vi "Return Black Start Status.vi"(4 "Status":T1, 6 "error":string, 8 "error in (no error)":errorcluster, 10 "IED Name":string, 11 "SCADA in":refnum<class "SCADA.lvclass">) -> (0 "error out":errorcluster, 3 "SCADA out":refnum<class "SCADA.lvclass">)   [LabVIEW 2015, in "SCADA Core.lvlib" / "SCADA.lvclass"]
uses:
  SCADA.lvclass
  SCADA Abstract Messages/Black Start Status Msg/Black Start Status.ctl
  SCADA.lvclass/SCADA.ctl
  <vilib>/ActorFramework/Actor/Actor.lvclass/Actor.ctl
  Controls/Grid Mode.ctl
  <vilib>/ActorFramework/Actor/Actor.lvclass
  SCADA Abstract Messages/Black Start Status Msg/Black Start Status Msg.lvclass
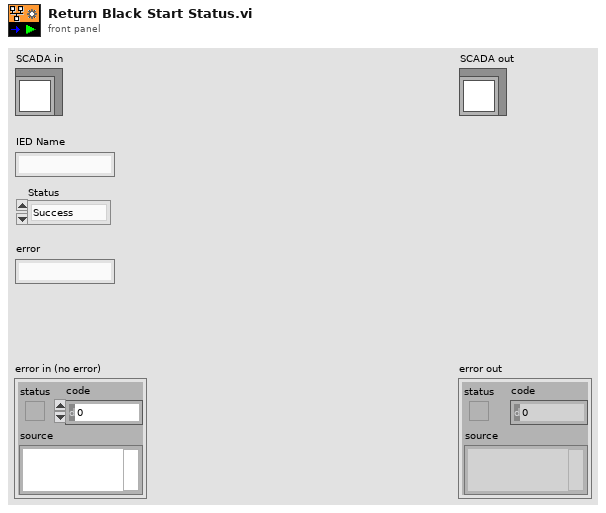
[diagram p1: front panel]
types:
  T1 = typedef "SCADA Core.lvlib/Black Start Status Msg.lvclass/Black Start Status.ctl" = enum16{"Success", "Failure"}
  T2 = typedef "SCADA Core.lvlib/SCADA.lvclass/Grid Mode.ctl" = enum16{"Off", "Grid Connected", "Islanded", "Synchronizing"}
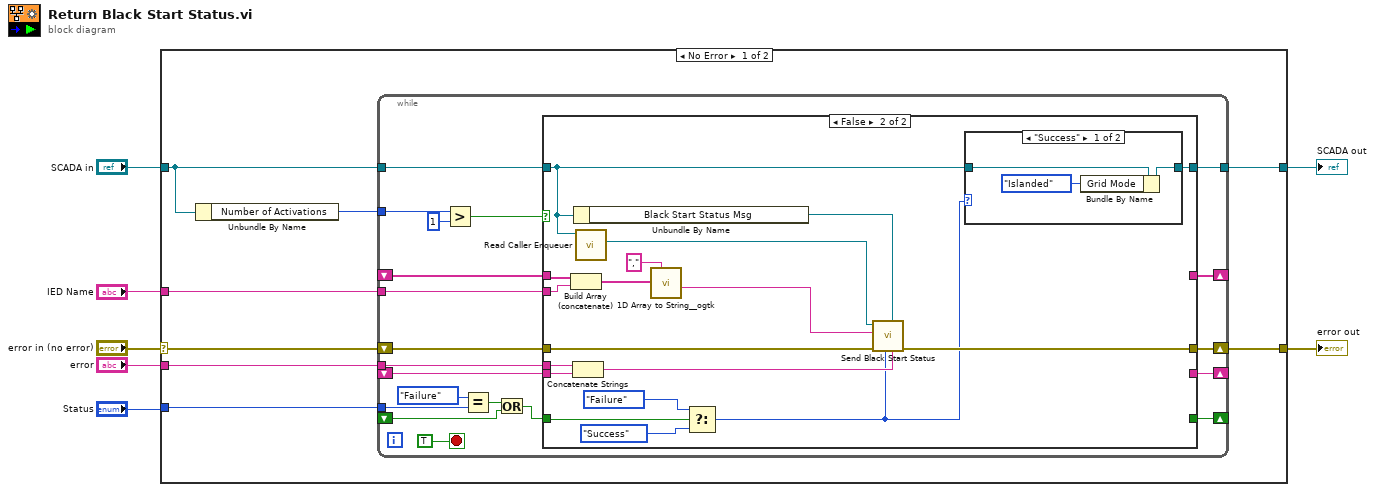
[diagram p0: block diagram]
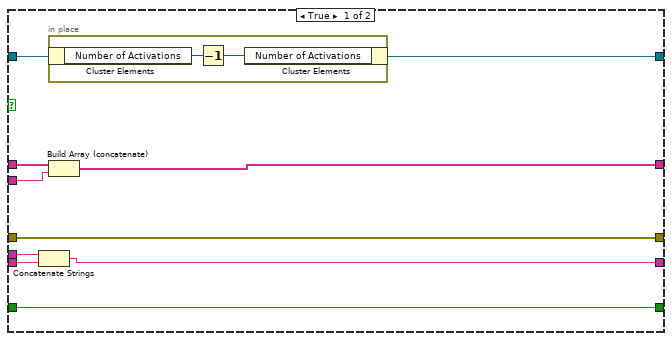
[diagram p2: hidden frame]
diagram:
  n1 = case shown="No Error" "error in (no error)" {
    selector: "error in (no error)" -> [w14 w71]
    tunnel: [w13 w71] -> w5
    tunnel: [w9 w70] -> w4
    tunnel: "SCADA in" -> [w10 w70]
    tunnel: "IED Name" -> [w15 _]
    tunnel: "error" -> [w12 _]
    tunnel: "Status" -> [w11 _]
    frame No Error {
      n2 = Unbundle By Name(w10) -> ("Number of Activations"=w8:i32)
      n3 = while {
        tunnel: w10 -> [w21]
        tunnel: w15 -> [w24]
        tunnel: w12 -> [w28]
        tunnel: w11 -> [w30]
        shift-right: [w34] -> _
        shift-left: _ -> [w31]
        shift-right: [w27] -> _
        shift-left: _ -> [w26]
        shift-right: [w23] -> _
        shift-left: _ -> [w22]
        shift-right: [w20] -> w13
        shift-left: w14 -> [w25]
        tunnel: [w19] -> w9
        tunnel: w8 -> [w17]
        stop <- TRUE stop-if-true
        n4 = Greater?(x=w17, y=1) -> (0:w16:bool)
        n5 = Equal?(x=Black_Start_Status."Failure" ("y"), y=w30) -> (x = y?=w33:bool)
        n6 = Or(x=w33, y=w31) -> (x .or. y?=w29:bool)
        n7 = case shown="False" w16 {
          tunnel: [w45 _] -> w34
          tunnel: w29 -> [w45 w63]
          tunnel: w28 -> [w44 w65]
          tunnel: [w43 _] -> w27
          tunnel: w26 -> [w42 w64]
          tunnel: w25 -> [w39 w58]
          tunnel: w24 -> [w36 w54]
          tunnel: [w41 _] -> w23
          tunnel: w22 -> [w40 w55]
          tunnel: w21 -> [w38 w50]
          tunnel: [w39 w56] -> w20
          tunnel: [w37 w49] -> w19
          frame True {
            n8 = Concatenate Strings(w44, w42) -> (w43:string)
            n9 = in-place {
              n10 = in-place-cluster #1(w38) -> ("Number of Activations"=w47:i32)
              n11 = Decrement(x=w47) -> (x-1=w46:i32)
              n12 = in-place-cluster #1("Number of Activations"=w46) -> (w37:refnum<class "SCADA.lvclass">)
            }
            n13 = Build Array (concatenate)(w40, w36) -> (w41:string[])
          }
          frame False {
            n14 = Build Array (concatenate)(w55, w54) -> (w53:string[])
            n15 = Concatenate Strings(w65, w64) -> (w57:string)
            n16 = Unbundle By Name(w50) -> ("Black Start Status Msg"=w60:refnum<class "Black Start Status Msg.lvclass">)
            n17 = call <vilib>:"Read Caller Enqueuer.vi"("Actor"=w50) -> ("Caller Enqueuer"=w59:refnum<class "Message Enqueuer.lvclass">)  [unwired: 10 in]
            n18 = call <userlib>:"1D Array to String__ogtk.vi"("delimiter (Tab)"=",", "Array of Strings"=w53) -> ("delimited string"=w51:string)  [unwired: 9 in]
            n19 = Select(t=Black_Start_Status."Failure" ("y"), s=w63, f=Black_Start_Status."Success" ("y")) -> (s? t:f=w48:T1)
            n20 = call "Send Black Start Status.vi"("error"=w57, "Black Start Status Msg"=w60, "Status"=w48, "error in (no error)"=w58, "Sequence"=w51, "Message Enqueuer in"=w59) -> ("error out"=w56:errorcluster)  [unwired: 4 in, 1 out]
            n21 = case shown="\"Success\"" w48 {
              tunnel: w50 -> [w68 w69]
              tunnel: [w67 w69] -> w49
              frame "Success" {
                n22 = Bundle By Name(cluster=w68, "Grid Mode"=Grid_Mode."Islanded") -> (w67:refnum<class "SCADA.lvclass">)
              }
              frame "Failure" {
              }
            }
          }
        }
      }
    }
    frame Error {
    }
  }
  "error out" <- w5
  "SCADA out" <- w4
